vi "Main.vi"() -> ()   [LabVIEW 2018] (continued)
            n2538 = call "S7_Read.vi"("TCP"=w7363, "DB #"=u16 20, "读取长度"=u16 1, "寄存器类型"=w7417, "起始地址"=u32 6, "数据类型"=w7413, "error in"=w7362) -> ("TCP"=w7412:refnum<k5>, "数据"=w7409:u32[], "error out"=w7403:errorcluster)  [unwired: 5 in, 1 out]
            n2539 = local read "ST10 Control Plat 5025303"() -> (w7387:string)
            n2540 = local read "ST10 Form Seal 5026859"() -> (w7390:string)
            n2541 = local read "ST10 Dowel Pin 5024532"() -> (w7389:string)
            n2542 = local read "ST10 Dowel Pin 5020281"() -> (w7388:string)
            n2543 = local read "ST10 Flange M0104918"() -> (w7386:string)
            n2544 = local read "ST10 Shaft M0102049"() -> (w7391:string)
            n2545 = Index Array(array=w7409) -> (element=w7408:u32)  [unwired: 1 in]
            n2546 = Equal?(x=w7408, y=u32 1) -> (x = y?=w7406:bool)
            n2547 = case shown="真" w7406 {
              tunnel: ["NG" "OK"] -> w7394
              frame False {
              }
              frame True {
              }
            }
            n2548 = Format Date/Time String(time format string (%c)="%Y-%m-%d" ("时间格式字符串(%c)")) -> (date/time string=w7396:string)  [unwired: 2 in]
            n2549 = Get Date/Time String() -> (time string=w7395:string)  [unwired: 3 in, 1 out]
            n2550 = Insert Into Array(array=string[] [] ("数组"), index=0 ("索引"), new element #1="101" ("新元素/子数组"), new element #2=w7394, new element #3=w7396, new element #4=w7395, new element #5=w7394, new element #6=w7391, new element #7=w7390, new element #8=w7389, new element #9=w7388, new element #10=w7387, new element #11=w7386, new element #12=w7371, new element #13=w7355, new element #14=w7354, new element #15=w7353, new element #16=w7352) -> (w7405:string[])
            n2551 = Enqueue Element(queue=w7404, element=w7405, error in (no error)=w7403) -> (error out=w7402:errorcluster)  [unwired: 1 in, 2 out]
            n2552 = property on="ST101数据读取（事件）" class="Bool (严格)"(error in=w7402, "Val(Sgnl)"=TRUE ("值(信号)")) -> (error out=w7392:errorcluster)  [unwired: 1 in, 1 out]
          }
          frame "数据保存回复" {
            w7436 = u8 132 items=["I/O (P)"=128, "Input (I)"=129, "Output (Q)"=130, "Bit Memory (M)"=131, "Data (DB)"=132, "Instance Data (DI)"=133, "Local Data (L)"=134, "Predecessor Local Data (VL)"=135] ("寄存器类型")
            w7437 = u16 1 items=["byte", "word", "Dword"] ("数据类型")
            n2553 = Index Array(array=w7430, index=0 ("索引")) -> (element=w7424:string)
            "数据保存请求回复101" <- w7424
            n2554 = Decimal String To Number(string=w7424, default (0L)=u32 0 ("默认(0 I32)")) -> (number=w7432:u32)  [unwired: 1 in, 1 out]
            n2555 = call "S7_Write.vi"("TCP"=w7431, "寄存器类型"=w7436, "DB #"=u16 20, "写入地址"=u32 4, "数据类型"=w7437, "写入数据"=w7432) -> ("TCP"=w7428:refnum<k5>, "error out"=w7429:errorcluster)  [unwired: 7 in, 1 out]
            n2556 = Bundle By Name(cluster=w7425, "数据保存1超时"=w7424) -> (w7423:T8)
            n2557 = call <vilib>:"Clear Errors.vi"("error in (no error)"=w7429) -> ("error out"=w7422:errorcluster)  [unwired: 5 in, 1 out]
          }
          frame "-----------------" {
          }
          frame "读扫码请求2" {
            w7457 = u8 132 items=["I/O (P)"=128, "Input (I)"=129, "Output (Q)"=130, "Bit Memory (M)"=131, "Data (DB)"=132, "Instance Data (DI)"=133, "Local Data (L)"=134, "Predecessor Local Data (VL)"=135] ("寄存器类型")
            w7456 = u16 1 items=["byte", "word", "Dword"] ("数据类型")
            w7465 = u16 0 items=["byte", "word", "Dword"] ("数据类型")
            w7467 = u8 132 items=["I/O (P)"=128, "Input (I)"=129, "Output (Q)"=130, "Bit Memory (M)"=131, "Data (DB)"=132, "Instance Data (DI)"=133, "Local Data (L)"=134, "Predecessor Local Data (VL)"=135] ("寄存器类型")
            n2558 = Unbundle By Name(w7449) -> ("看门狗"=w7454:string)
            n2559 = Decimal String To Number(string=w7454) -> (number=w7453:i32)  [unwired: 2 in, 1 out]
            n2560 = Equal?(x=w7453, y=0) -> (x = y?=w7451:bool)
            n2561 = case shown="假" w7451 {
              tunnel: [0 ("y") 1 ("y")] -> w7444
              frame False {
              }
              frame True {
              }
            }
            n2562 = local write "10"(w7444) -> ()
            n2563 = call "S7_Write.vi"("TCP"=w7447, "寄存器类型"=w7457, "DB #"=u16 20, "写入地址"=u32 22, "数据类型"=w7456, "写入数据"=w7444) -> ("TCP"=w7446:refnum<k5>, "error out"=w7445:errorcluster)  [unwired: 7 in, 1 out]
            n2564 = Number To Decimal String(number=w7444) -> (decimal integer string=w7450:string)  [unwired: 1 in]
            n2565 = Bundle By Name(cluster=w7449, "看门狗"=w7450) -> (w7448:T8)
            n2566 = call "S7_Read.vi"("TCP"=w7446, "DB #"=u16 20, "读取长度"=u16 1, "寄存器类型"=w7467, "起始地址"=u32 0, "数据类型"=w7465, "error in"=w7445) -> ("TCP"=w7463:refnum<k5>, "数据"=w7487:u32[], "error out"=w7464:errorcluster)  [unwired: 5 in, 1 out]
            n2567 = Index Array(array=w7487, index=0 ("索引")) -> (element=w7486:u32)
            n2568 = Number To Boolean Array(number=w7486) -> (Boolean array=w7485:bool[])
            n2569 = Index Array(array=w7485, index=2 ("索引")) -> (element=w7460:bool)
            "ST102扫码请求" <- w7460
            n2570 = Unbundle By Name(w7448) -> ("扫码2超时"=w7477:string)
            n2571 = Not Equal?(x=w7477, y="999") -> (x != y?=w7478:bool)
            n2572 = Not(x=w7478) -> (.not. x?=w7479:bool)
            n2573 = call <vilib>:"Boolean Crossing PtByPt.vi"("direction"=enum16{"either", "false-true", "true-false"}."false-true", "input"=w7460) -> ("crossing"=w7484:bool)  [unwired: 1 in]
            n2574 = call <vilib>:"Boolean Crossing PtByPt.vi"("direction"=enum16{"either", "false-true", "true-false"}."true-false", "input"=w7460) -> ("crossing"=w7483:bool)  [unwired: 1 in]
            n2575 = call "已用时间"("Reset"=w7479) -> ("Time has Elapsed"=w7480:bool)  [unwired: 11 in, 7 out]
            n2576 = Insert Into Array(array=bool[] [] ("数组"), index=0 ("索引"), new element #1=w7484, new element #2=w7483) -> (w7482:bool[])
            n2577 = Boolean Array To Number(Boolean array=w7482) -> (number=w7481:u32)
            n2578 = case shown="2" w7481 {
              tunnel: [cluster{"Data":string[], "State":T1} {"Data"=[], "State"=enum."读数据保存请求2"} ("元素") w7495 w7498] -> w7462
              tunnel: w7461 -> [_ w7496 w7499]
              frame 0, Default {
              }
              frame 1 {
                w7495 = cluster{"Data":string[], "State":T1} {"Data"=[], "State"=enum."读二维码2"} ("元素")
                n2579 = Enqueue Element(queue=w7496, element=w7495, timeout in ms (-1)=10 ("超时毫秒(-1)")) -> ()  [unwired: 1 in, 3 out]
              }
              frame 2 {
                w7498 = cluster{"Data":string[], "State":T1} {"Data"=["999"], "State"=enum."扫码回复2"} ("元素")
                n2580 = Enqueue Element(queue=w7499, element=w7498, timeout in ms (-1)=10 ("超时毫秒(-1)")) -> ()  [unwired: 1 in, 3 out]
              }
            }
            n2581 = case shown="真" w7480 {
              tunnel: w7461 -> [_ w7491]
              frame False {
              }
              frame True {
                n2582 = Enqueue Element(queue=w7491, element=cluster{"Data":string[], "State":T1} {"Data"=["999"], "State"=enum."扫码回复2"} ("元素"), timeout in ms (-1)=10 ("超时毫秒(-1)")) -> ()  [unwired: 1 in, 3 out]
              }
            }
          }
          frame "读二维码2" {
            w7511 = u16 0 items=["byte", "word", "Dword"] ("数据类型")
            w7513 = u8 132 items=["I/O (P)"=128, "Input (I)"=129, "Output (Q)"=130, "Bit Memory (M)"=131, "Data (DB)"=132, "Instance Data (DI)"=133, "Local Data (L)"=134, "Predecessor Local Data (VL)"=135] ("寄存器类型")
            n2583 = call "S7_Read.vi"("TCP"=w7510, "DB #"=u16 20, "读取长度"=u16 17, "寄存器类型"=w7513, "起始地址"=u32 42, "数据类型"=w7511) -> ("TCP"=w7508:refnum<k5>, "数据"=w7516:u32[], "error out"=w7518:errorcluster)  [unwired: 6 in, 1 out]
            n2584 = To Unsigned Word Integer(number=w7516) -> (unsigned 16bit integer=w7517:u16[])
            n2585 = call "还原为字符串.vi"("error in (no error)"=w7518, "输入数组"=w7517) -> ("error out"=w7502:errorcluster, "字符串"=w7503:string)  [unwired: 8 in]
            n2586 = Match Pattern(string=w7503, regular expression=" " ("正则表达式")) -> (before substring=w7500:string)  [unwired: 1 in, 3 out]
            n2587 = flat-sequence {
              tunnel: w7502 -> [w7520]
              tunnel: [w7520] -> w7501
              tunnel: w7500 -> [w7519]
              tunnel: [w7522] -> w7507
              tunnel: w7501 -> [w7521]
              frame #0 {
                "102 二维码" <- w7519
              }
              frame #1 {
                n2588 = property on="ST102扫码请求（事件）" class="Bool (严格)"(error in=w7521, "Val(Sgnl)"=TRUE ("值(信号)")) -> (error out=w7522:errorcluster)  [unwired: 1 in, 1 out]
              }
            }
          }
          frame "扫码回复2" {
            n2589 = Array Size(array=w7531) -> (size(s)=w7534:i32)
            n2590 = case shown="3, 默认" w7534 {
              tunnel: w7532 -> [w7547 w7570]
              tunnel: [w7538 w7572] -> w7528
              tunnel: [w7537 w7571] -> w7527
              tunnel: w7531 -> [w7536 w7569]
              tunnel: [w7535 w7567] -> w7529
              frame 3, Default {
                w7550 = u8 132 items=["I/O (P)"=128, "Input (I)"=129, "Output (Q)"=130, "Bit Memory (M)"=131, "Data (DB)"=132, "Instance Data (DI)"=133, "Local Data (L)"=134, "Predecessor Local Data (VL)"=135] ("寄存器类型")
                w7549 = u16 1 items=["byte", "word", "Dword"] ("数据类型")
                w7557 = u8 132 items=["I/O (P)"=128, "Input (I)"=129, "Output (Q)"=130, "Bit Memory (M)"=131, "Data (DB)"=132, "Instance Data (DI)"=133, "Local Data (L)"=134, "Predecessor Local Data (VL)"=135] ("寄存器类型")
                w7558 = u16 1 items=["byte", "word", "Dword"] ("数据类型")
                w7563 = u8 132 items=["I/O (P)"=128, "Input (I)"=129, "Output (Q)"=130, "Bit Memory (M)"=131, "Data (DB)"=132, "Instance Data (DI)"=133, "Local Data (L)"=134, "Predecessor Local Data (VL)"=135] ("寄存器类型")
                w7562 = u16 1 items=["byte", "word", "Dword"] ("数据类型")
                n2591 = Index Array(array=w7536) -> (element #1=w7535:string, element #2=w7543:string, element #3=w7542:string)  [unwired: 3 in]
                n2592 = Equal?(x=w7542, y="OK") -> (x = y?=w7540:bool)
                n2593 = Decimal String To Number(string=w7543, default (0L)=u32 0 ("默认(0 I32)")) -> (number=w7544:u32)  [unwired: 1 in, 1 out]
                n2594 = case shown="真" w7540 {
                  tunnel: [u32 2 ("写入数据") u32 1 ("写入数据")] -> w7539
                  frame False {
                  }
                  frame True {
                  }
                }
                n2595 = call "S7_Write.vi"("TCP"=w7547, "寄存器类型"=w7563, "DB #"=u16 20, "写入地址"=u32 18, "数据类型"=w7562, "写入数据"=w7544) -> ("TCP"=w7554:refnum<k5>, "error out"=w7555:errorcluster)  [unwired: 7 in, 1 out]
                n2596 = call "S7_Write.vi"("TCP"=w7554, "寄存器类型"=w7557, "DB #"=u16 20, "写入地址"=u32 20, "数据类型"=w7558, "写入数据"=w7539, "error in"=w7555) -> ("TCP"=w7546:refnum<k5>, "error out"=w7545:errorcluster)  [unwired: 6 in, 1 out]
                n2597 = Decimal String To Number(string=w7535, default (0L)=u32 0 ("默认(0 I32)")) -> (number=w7553:u32)  [unwired: 1 in, 1 out]
                n2598 = call "S7_Write.vi"("TCP"=w7546, "寄存器类型"=w7550, "DB #"=u16 20, "写入地址"=u32 14, "数据类型"=w7549, "写入数据"=w7553, "error in"=w7545) -> ("TCP"=w7538:refnum<k5>, "error out"=w7537:errorcluster)  [unwired: 6 in, 1 out]
              }
              frame 1 {
                w7575 = u8 132 items=["I/O (P)"=128, "Input (I)"=129, "Output (Q)"=130, "Bit Memory (M)"=131, "Data (DB)"=132, "Instance Data (DI)"=133, "Local Data (L)"=134, "Predecessor Local Data (VL)"=135] ("寄存器类型")
                w7574 = u16 1 items=["byte", "word", "Dword"] ("数据类型")
                n2599 = Index Array(array=w7569, index=0 ("索引")) -> (element=w7567:string)
                n2600 = Decimal String To Number(string=w7567, default (0L)=u32 0 ("默认(0 I32)")) -> (number=w7578:u32)  [unwired: 1 in, 1 out]
                n2601 = call "S7_Write.vi"("TCP"=w7570, "寄存器类型"=w7575, "DB #"=u16 20, "写入地址"=u32 14, "数据类型"=w7574, "写入数据"=w7578) -> ("TCP"=w7572:refnum<k5>, "error out"=w7571:errorcluster)  [unwired: 7 in, 1 out]
              }
            }
            "扫码请求回复102" <- w7529
            n2602 = Bundle By Name(cluster=w7533, "扫码2超时"=w7529) -> (w7526:T8)
            n2603 = call <vilib>:"Clear Errors.vi"("error in (no error)"=w7527) -> ("error out"=w7524:errorcluster)  [unwired: 5 in, 1 out]
          }
          frame "-- --------------" {
          }
          frame "读数据保存请求2" {
            w7591 = u16 0 items=["byte", "word", "Dword"] ("数据类型")
            w7593 = u8 132 items=["I/O (P)"=128, "Input (I)"=129, "Output (Q)"=130, "Bit Memory (M)"=131, "Data (DB)"=132, "Instance Data (DI)"=133, "Local Data (L)"=134, "Predecessor Local Data (VL)"=135] ("寄存器类型")
            n2604 = call "S7_Read.vi"("TCP"=w7590, "DB #"=u16 20, "读取长度"=u16 1, "寄存器类型"=w7593, "起始地址"=u32 0, "数据类型"=w7591) -> ("TCP"=w7588:refnum<k5>, "数据"=w7614:u32[], "error out"=w7587:errorcluster)  [unwired: 6 in, 1 out]
            n2605 = Index Array(array=w7614, index=0 ("索引")) -> (element=w7613:u32)
            n2606 = Number To Boolean Array(number=w7613) -> (Boolean array=w7612:bool[])
            n2607 = Unbundle By Name(w7589) -> ("数据保存2超时"=w7603:string)
            n2608 = Index Array(array=w7612, index=3 ("索引")) -> (element=w7607:bool)
            "ST102数据读取" <- w7607
            n2609 = Not Equal?(x=w7603, y="999") -> (x != y?=w7604:bool)
            n2610 = Not(x=w7604) -> (.not. x?=w7605:bool)
            n2611 = call <vilib>:"Boolean Crossing PtByPt.vi"("direction"=enum16{"either", "false-true", "true-false"}."false-true", "input"=w7607) -> ("crossing"=w7608:bool)  [unwired: 1 in]
            n2612 = call <vilib>:"Boolean Crossing PtByPt.vi"("direction"=enum16{"either", "false-true", "true-false"}."true-false", "input"=w7607) -> ("crossing"=w7609:bool)  [unwired: 1 in]
            n2613 = call "已用时间2"("Reset"=w7605) -> ("Time has Elapsed"=w7606:bool)  [unwired: 11 in, 7 out]
            n2614 = Insert Into Array(array=bool[] [] ("数组"), index=0 ("索引"), new element #1=w7608, new element #2=w7609) -> (w7610:bool[])
            n2615 = Boolean Array To Number(Boolean array=w7610) -> (number=w7611:u32)
            n2616 = case shown="1" w7611 {
              tunnel: [cluster{"Data":string[], "State":T1} {"Data"=[], "State"=enum."看门狗"} ("元素") w7620 w7622] -> w7584
              tunnel: w7586 -> [_ w7621 w7623]
              frame 0, Default {
              }
              frame 1 {
                w7620 = cluster{"Data":string[], "State":T1} {"Data"=[], "State"=enum."读数据2"} ("元素")
                n2617 = Enqueue Element(queue=w7621, element=w7620, timeout in ms (-1)=10 ("超时毫秒(-1)")) -> ()  [unwired: 1 in, 3 out]
              }
              frame 2 {
                w7622 = cluster{"Data":string[], "State":T1} {"Data"=["999"], "State"=enum."数据保存回复2"} ("元素")
                n2618 = Enqueue Element(queue=w7623, element=w7622, timeout in ms (-1)=10 ("超时毫秒(-1)")) -> ()  [unwired: 1 in, 3 out]
              }
            }
            n2619 = case shown="真" w7606 {
              tunnel: w7586 -> [_ w7616]
              frame False {
              }
              frame True {
                n2620 = Enqueue Element(queue=w7616, element=cluster{"Data":string[], "State":T1} {"Data"=["999"], "State"=enum."数据保存回复2"} ("元素"), timeout in ms (-1)=10 ("超时毫秒(-1)")) -> ()  [unwired: 1 in, 3 out]
              }
            }
          }
          frame "读数据2" {
            w7634 = u16 1 items=["byte", "word", "Dword"] ("数据类型")
            w7636 = u8 132 items=["I/O (P)"=128, "Input (I)"=129, "Output (Q)"=130, "Bit Memory (M)"=131, "Data (DB)"=132, "Instance Data (DI)"=133, "Local Data (L)"=134, "Predecessor Local Data (VL)"=135] ("寄存器类型")
            n2621 = call "S7_Read.vi"("TCP"=w7629, "DB #"=u16 20, "读取长度"=u16 1, "寄存器类型"=w7636, "起始地址"=u32 12, "数据类型"=w7634) -> ("TCP"=w7633:refnum<k5>, "数据"=w7649:u32[], "error out"=w7627:errorcluster)  [unwired: 6 in, 1 out]
            n2622 = Index Array(array=w7649) -> (element=w7648:u32)  [unwired: 1 in]
            n2623 = Equal?(x=w7648, y=u32 1) -> (x = y?=w7647:bool)
            n2624 = case shown="真" w7647 {
              tunnel: ["NG" "OK"] -> w7644
              frame False {
              }
              frame True {
              }
            }
            n2625 = Format Date/Time String(time format string (%c)="%Y-%m-%d" ("时间格式字符串(%c)")) -> (date/time string=w7646:string)  [unwired: 2 in]
            n2626 = Get Date/Time String() -> (time string=w7645:string)  [unwired: 3 in, 1 out]
            n2627 = Insert Into Array(array=string[] [] ("数组"), index=0 ("索引"), new element #1="102" ("新元素/子数组"), new element #2=w7644, new element #3=w7646, new element #4=w7645, new element #5=w7644) -> (w7625:string[])
            n2628 = flat-sequence {
              tunnel: w7627 -> [w7651]
              tunnel: [w7651] -> w7626
              tunnel: w7625 -> [w7650]
              tunnel: [w7654] -> w7628
              tunnel: w7626 -> [w7652]
              frame #0 {
                "102读取数据" <- w7650
              }
              frame #1 {
                n2629 = property on="ST102数据读取（事件）" class="Bool (严格)"(error in=w7652, "Val(Sgnl)"=TRUE ("值(信号)")) -> (error out=w7654:errorcluster)  [unwired: 1 in, 1 out]
              }
            }
          }
          frame "数据保存回复2" {
            w7669 = u8 132 items=["I/O (P)"=128, "Input (I)"=129, "Output (Q)"=130, "Bit Memory (M)"=131, "Data (DB)"=132, "Instance Data (DI)"=133, "Local Data (L)"=134, "Predecessor Local Data (VL)"=135] ("寄存器类型")
            w7666 = u16 1 items=["byte", "word", "Dword"] ("数据类型")
            n2630 = Index Array(array=w7663, index=0 ("索引")) -> (element=w7672:string)
            "数据保存请求回复102" <- w7672
            n2631 = Decimal String To Number(string=w7672, default (0L)=u32 0 ("默认(0 I32)")) -> (number=w7673:u32)  [unwired: 1 in, 1 out]
            n2632 = call "S7_Write.vi"("TCP"=w7665, "寄存器类型"=w7669, "DB #"=u16 20, "写入地址"=u32 16, "数据类型"=w7666, "写入数据"=w7673) -> ("TCP"=w7661:refnum<k5>, "error out"=w7662:errorcluster)  [unwired: 7 in, 1 out]
            n2633 = Bundle By Name(cluster=w7664, "数据保存2超时"=w7672) -> (w7659:T8)
            n2634 = call <vilib>:"Clear Errors.vi"("error in (no error)"=w7662) -> ("error out"=w7657:errorcluster)  [unwired: 5 in, 1 out]
          }
          frame "------------" {
          }
          frame "错误" {
            n2635 = Flush Queue(queue=w7681) -> ()  [unwired: 1 in, 3 out]
            n2636 = Flush Queue(queue=w7680) -> ()  [unwired: 1 in, 3 out]
            n2637 = call "S7_Close.vi"("TCP Connection Ref"=w7684) -> ("error out"=w7682:errorcluster)  [unwired: 10 in]
            n2638 = call <vilib>:"Clear Errors.vi"("error in (no error)"=w7682) -> ()  [unwired: 5 in, 2 out]
          }
          frame "退出" {
            n2639 = Release Queue(queue=w7693) -> ()  [unwired: 2 in, 3 out]
            n2640 = Release Queue(queue=w7692) -> ()  [unwired: 2 in, 3 out]
            n2641 = call "S7_Close.vi"("TCP Connection Ref"=w7691) -> ("error out"=w7690:errorcluster)  [unwired: 10 in]
          }
          frame "看门狗" {
            w7706 = "\r" ("正则表达式")
            w7716 = u16 0 items=["byte", "word", "Dword"] ("数据类型")
            w7718 = u8 132 items=["I/O (P)"=128, "Input (I)"=129, "Output (Q)"=130, "Bit Memory (M)"=131, "Data (DB)"=132, "Instance Data (DI)"=133, "Local Data (L)"=134, "Predecessor Local Data (VL)"=135] ("寄存器类型")
            w7737 = u8 132 items=["I/O (P)"=128, "Input (I)"=129, "Output (Q)"=130, "Bit Memory (M)"=131, "Data (DB)"=132, "Instance Data (DI)"=133, "Local Data (L)"=134, "Predecessor Local Data (VL)"=135] ("寄存器类型")
            w7736 = u16 1 items=["byte", "word", "Dword"] ("数据类型")
            n2642 = Unbundle By Name(w7727) -> ("看门狗"=w7733:string)
            n2643 = Decimal String To Number(string=w7733) -> (number=w7732:i32)  [unwired: 2 in, 1 out]
            n2644 = Equal?(x=w7732, y=0) -> (x = y?=w7730:bool)
            n2645 = case shown="假" w7730 {
              tunnel: [0 ("y") 1 ("y")] -> w7729
              frame False {
              }
              frame True {
              }
            }
            "10" <- w7729
            n2646 = call "S7_Write.vi"("TCP"=w7734, "寄存器类型"=w7737, "DB #"=u16 20, "写入地址"=u32 22, "数据类型"=w7736, "写入数据"=w7729) -> ("TCP"=w7715:refnum<k5>, "error out"=w7714:errorcluster)  [unwired: 7 in, 1 out]
            n2647 = Number To Decimal String(number=w7729) -> (decimal integer string=w7728:string)  [unwired: 1 in]
            n2648 = Bundle By Name(cluster=w7727, "看门狗"=w7728) -> (w7726:T8)
            n2649 = call "S7_Read.vi"("TCP"=w7715, "DB #"=u16 20, "读取长度"=u16 120, "寄存器类型"=w7718, "起始地址"=u32 60, "数据类型"=w7716, "error in"=w7714) -> ("TCP"=w7699:refnum<k5>, "数据"=w7724:u32[], "error out"=w7697:errorcluster)  [unwired: 5 in, 1 out]
            n2650 = To Unsigned Word Integer(number=w7724) -> (unsigned 16bit integer=w7725:u16[])
            n2651 = call "还原为字符串.vi"("输入数组"=w7725) -> ("字符串"=w7723:string)  [unwired: 9 in, 1 out]
            n2652 = for {
              N: 8 -> [_]
              tunnel: w7723 -> [w7757]
              tunnel: [w7756] -> w7713 mode=indexing
              shift-right: [w7752] -> _
              shift-left: 0 ("长度（剩余）") -> [w7754]
              n2653 = String Subset(string=w7757, offset (0)=w7754, length (rest)=20 ("长度（剩余）")) -> (substring=w7756:string)
              n2654 = Add(x=w7754, y=20) -> (x+y=w7752:i32)
            }
            n2655 = Index Array(array=w7713) -> (element #1=w7712:string, element #2=w7711:string, element #3=w7710:string, element #4=w7709:string, element #5=w7708:string, element #6=w7707:string)  [unwired: 6 in]
            n2656 = Match Pattern(string=w7712, regular expression=w7706) -> (before substring=→"ST10 Shaft M0102049":string)  [unwired: 1 in, 3 out]
            n2657 = Match Pattern(string=w7711, regular expression=w7706) -> (before substring=→"ST10 Form Seal 5026859":string)  [unwired: 1 in, 3 out]
            n2658 = Match Pattern(string=w7710, regular expression=w7706) -> (before substring=→"ST10 Dowel Pin 5024532":string)  [unwired: 1 in, 3 out]
            n2659 = Match Pattern(string=w7709, regular expression=w7706) -> (before substring=→"ST10 Dowel Pin 5020281":string)  [unwired: 1 in, 3 out]
            n2660 = Match Pattern(string=w7708, regular expression=w7706) -> (before substring=→"ST10 Control Plat 5025303":string)  [unwired: 1 in, 3 out]
            n2661 = Match Pattern(string=w7707, regular expression=w7706) -> (before substring=→"ST10 Flange M0104918":string)  [unwired: 1 in, 3 out]
            n2662 = disable-structure shown="启用" {
              disable-tunnel: w7699 -> [w7741 w7745]
              disable-tunnel: [w7741 w7748] -> w7698
              disable-tunnel: w7697 -> [w7742 w7746]
              disable-tunnel: [w7742 w7747] -> w7696
              frame Disabled {
              }
              frame Enabled {
                w7750 = u8 132 items=["I/O (P)"=128, "Input (I)"=129, "Output (Q)"=130, "Bit Memory (M)"=131, "Data (DB)"=132, "Instance Data (DI)"=133, "Local Data (L)"=134, "Predecessor Local Data (VL)"=135] ("寄存器类型")
                w7744 = u16 1 items=["byte", "word", "Dword"] ("数据类型")
                n2663 = local read "80产品型号"() -> (w7743:u32)
                n2664 = call "S7_Write.vi"("TCP"=w7745, "寄存器类型"=w7750, "DB #"=u16 20, "写入地址"=u32 236, "数据类型"=w7744, "写入数据"=w7743, "error in"=w7746) -> ("TCP"=w7748:refnum<k5>, "error out"=w7747:errorcluster)  [unwired: 6 in, 1 out]
              }
            }
          }
        }
      }
    }
  }
